vi "SetUpLeCroy930xx.vi"(6 "Therapy (T)":bool, 7 "Therapy VISA session in":refnum<visa-resource-name>, 8 "33250(T)/33120(F)":bool=TRUE, 11 "VISA session":refnum<visa-resource-name>) -> (1 "Equivalent delay\ndistance (mm)":dbl=1.5 format="%.2f", 2 "RF data Out":T2 {"Delay (micro s)" format="%.2f"})   [LabVIEW 2022 SP3]
uses:
  Motion Controllers/-MotionRoutines/MotionGlobals.vi
  <vilib>/Analysis/NI_AALPro.lvlib
  <vilib>/Utility/file.llb/Write To Spreadsheet File (DBL).vi
  <vilib>/Analysis/NI_AALBase.lvlib
  <vilib>/Analysis/baseanly.llb/Mean (DBL).vi
panel:
  in  "Grab Settings":bool
  in  "Save trace?":bool
  out "Lines in burst":i32=1 min=1 max=50000 step=1
  in  "cycles (f), time(t)":bool=TRUE
  in  "Set Panametrics":bool
  out "Scope Delay (ms)":dbl=1.5 format="%.2f"
  in  "go to scan type":bool
  in  "Therapy Burst Set Up":T1={"Therapy Set Up"={"Burst time (ms)"=1.0, "Frequency (MHz)"=1.0, "Amplitude (mV)"=10.0}, "Divide prf by"=1, "Therapy Delay (ms) "=0.0, "Turn off therapy (T)"=TRUE} {"Therapy Delay (ms)" format="%.2f"; "Therapy Set Up"."Amplitude (mV)" min=10.0 max=1000.0 format="%.2f"; "Therapy Set Up"."Frequency (MHz)" format="%.4f"; "Therapy Set Up"."Burst time (ms)" min=1 max=50000 step=1 format="%.3f"}
  in  "ExitSendCmd":bool
  out "Time scale per Div":i32(ring)=3 items=["100 ns", "200 ns", "500 ns", "1 micros", "2 micros", "5 micros", "10 micros", "20 micros", "50 micros", "100 micros", "200 micros", "500 micros", "1 ms", "2 ms", "5 ms", "10 ms", "20 ms", "50 ms", "100 ms", "200 ms"]
  out "Waveform\nGraph":cluster{i32, dbl, dbl[]}(graph)
  in  "Trigger Settings":T3={"Source"=1, "Coupling"=0, "Slope"=0, "Level (mV)"=1000.0} {"Slope" items=["Positive", "Negative"]; "Level (mV)" format="%.2f"; "Coupling" items=["DC 1 MOhm", "AC 1 MOhm", "DC 50 Ohm", "AC 50 Ohm"]; "Source" items=["Chan 1", "External"]}
  in  "RF data Sampling":T4={"Sampling Rate"=5, "Ref Delay (ms)"=0.0, "rf points per line"=2048} {"Ref Delay (ms)" format="%.2f"}
  # "Digitizer Settings"
  # "Set Up trace on Scope, then select Grab Settings to verify trace is captured."
  # "Need to autoscale if viewing spectrum. Yellow curser used for additional delay.\nRF data is captured between yellow and red lines."
  # "© 2000-2002 Riverside Research Institute"
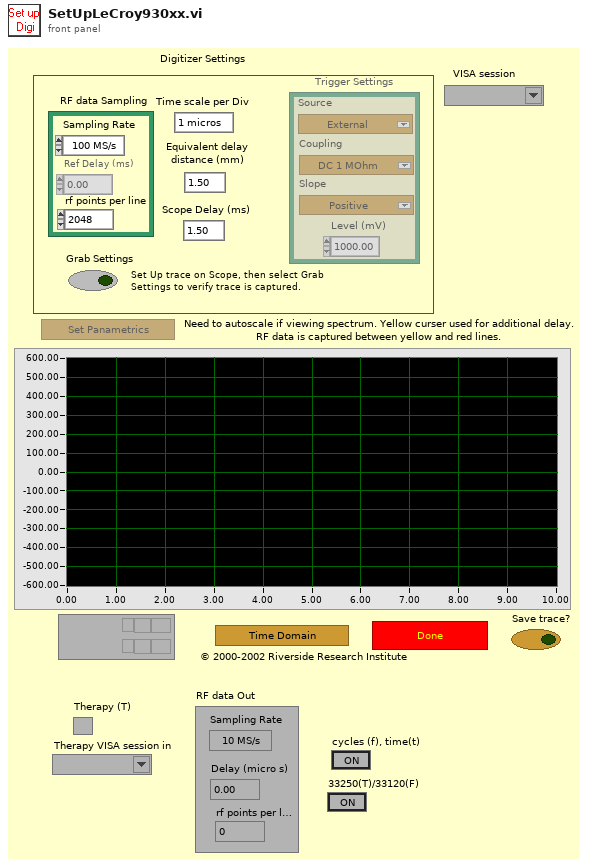
[diagram p1: front panel]
types:
  T1 = cluster{"Therapy Set Up":cluster{"Burst time (ms)":sgl, "Frequency (MHz)":dbl, "Amplitude (mV)":dbl}, "Divide prf by":i32, "Therapy Delay (ms) ":dbl, "Turn off therapy (T)":bool}
  T2 = cluster{"Sampling Rate":u16, "Delay (micro s)":dbl, "rf points per line":u16}
  T3 = cluster{"Source":u16, "Coupling":u16, "Slope":u16, "Level (mV)":dbl}
  T4 = cluster{"Sampling Rate":u16, "Ref Delay (ms)":dbl, "rf points per line":u16}
  T5 = cluster{"Burst time (ms)":sgl, "Frequency (MHz)":dbl, "Amplitude (mV)":dbl}
  T6 = cluster{"t(0) (sec)":ext, "Delta t (sec)":dbl, "Amplitude Array (Volts)":sgl[]}
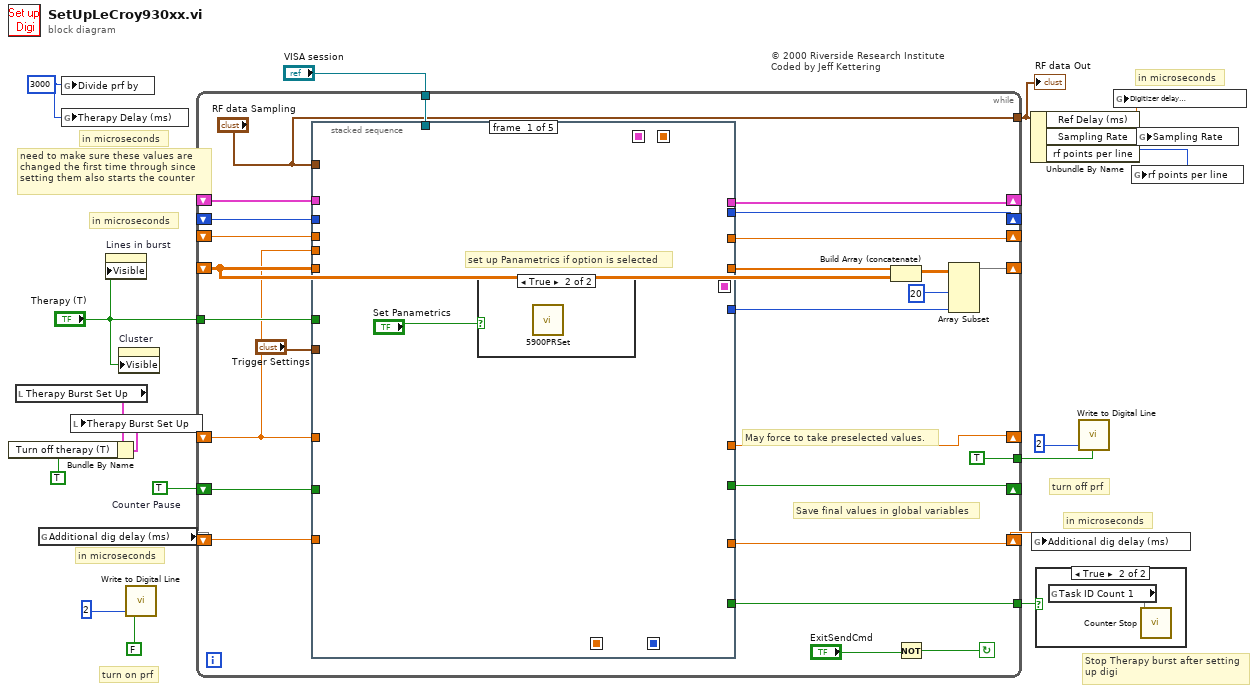
[diagram p0: block diagram]
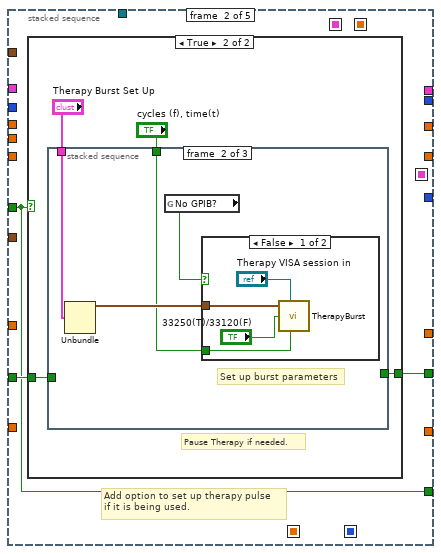
[diagram p3: hidden frame]
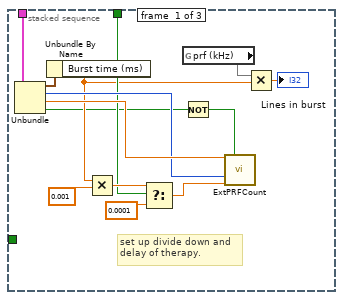
[diagram p5: hidden frame]
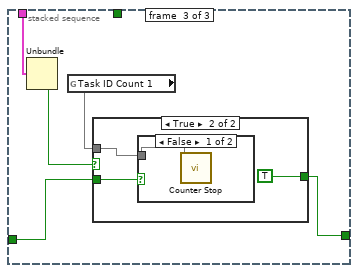
[diagram p7: hidden frame]
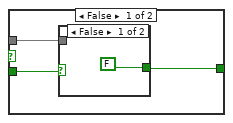
[diagram p8: hidden frame]
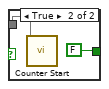
[diagram p9: hidden frame]
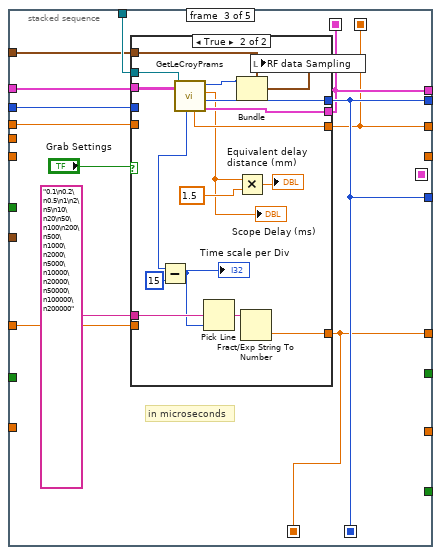
[diagram p11: hidden frame]
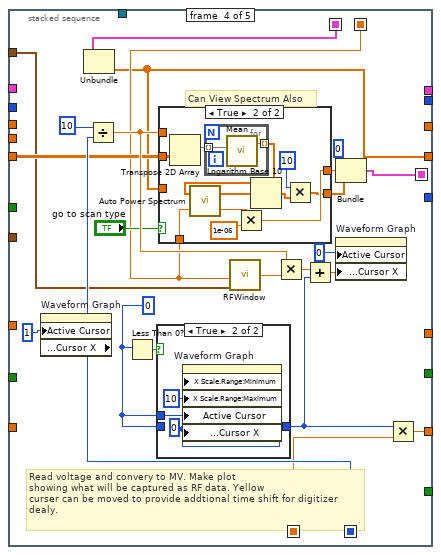
[diagram p13: hidden frame]
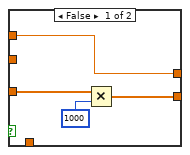
[diagram p15: hidden frame]
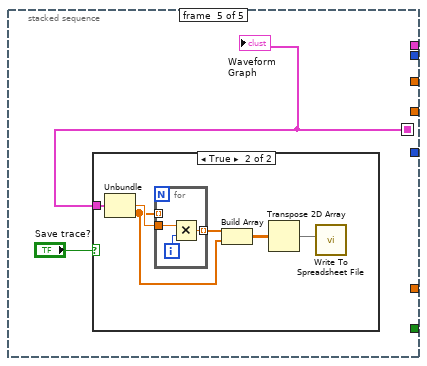
[diagram p16: hidden frame]
diagram:
  w17 = 3000
  w18 = TRUE  # Counter Pause
  # "turn on prf"
  # "turn off prf"
  # "© 2000 Riverside Research Institute\nCoded by Jeff Kettering"
  # "Stop Therapy burst after setting\nup digi"
  # "in microseconds"
  # "in microseconds"
  # "in microseconds"
  # "in microseconds"
  # "in microseconds"
  # "need to make sure these values are\nchanged the first time through since\nsetting them also starts the counter"
  n1 = local read "Therapy Burst Set Up"() -> (w10:T1)
  n2 = Bundle By Name(cluster=w10, "Turn off therapy (T)"=TRUE) -> (w9:T1)
  n3 = global read "MotionGlobals.vi" "Additional dig delay (ms)"() -> (w12)
  n4 = global write "MotionGlobals.vi" "Divide prf by"(w17) -> ()
  n5 = global write "MotionGlobals.vi" "Therapy Delay (ms)"(w17) -> ()
  n6 = local write "Therapy Burst Set Up"(w9) -> ()
  n7 = property on="Lines in burst" class="DigNum (strict)"("Visible"="Therapy (T)") -> ()  [unwired: 2 in, 2 out]
  n8 = property on="Cluster" class="Clust (strict)"("Visible"="Therapy (T)") -> ()  [unwired: 2 in, 2 out]
  n9 = call <vilib>:"Write to Digital Line.vi"("line"=2, "line state"=FALSE) -> ()  [unwired: 7 in]
  n10 = while {
    tunnel: [TRUE] -> w3
    tunnel: [w30] -> w7
    shift-left: _ -> [w35]
    shift-right: [w33] -> _
    shift-left: w12 -> [w38]
    shift-right: [w37] -> w11
    tunnel: ["RF data Sampling"] -> w14
    shift-left: w18 -> [w40]
    shift-right: [w39] -> _
    tunnel: "Therapy (T)" -> [w41]
    tunnel: "VISA session" -> [w28]
    shift-right: [w26] -> _
    shift-left: _ -> [w24]
    shift-right: [w27] -> _
    shift-left: _ -> [w22]
    shift-right: [w25] -> _
    shift-left: _ -> [w23]
    shift-right: [w20] -> _
    shift-left: _ -> [w21]
    stop <- w42 continue-if-true
    # "May force to take preselected values."
    # "Save final values in global variables"
    n11 = stacked-sequence {
      seq-local: [_ _ w99 _ _] -> [_ _ _ w141 _]
      seq-local: [_ _ w92 _ _] -> [_ _ _ w137 _]
      seq-local: [_ _ _ w128 _] -> [_ _ _ _ w167]
      seq-local: [_ _ w98 _ _] -> [_ _ _ w126 _]
      seq-local: [_ _ w97 _ _] -> [_ _ _ w127 _]
      tunnel: "RF data Sampling" -> [_ _ w91 w130 _]
      tunnel: "Trigger Settings" -> [_ _ _ _ _]
      tunnel: w41 -> [_ w46 _ _ _]
      tunnel: w40 -> [_ w48 _ _ _]
      tunnel: [_ w47 _ _ _] -> w39
      tunnel: w38 -> [_ _ _ _ _]
      tunnel: [_ _ _ w129 _] -> w37
      tunnel: w35 -> [_ _ _ w132 _]
      tunnel: [_ _ _ w125 _] -> w36
      tunnel: [_ _ w99 _ _] -> w32
      tunnel: [_ w46 _ _ _] -> w30
      tunnel: w28 -> [_ _ w101 _ _]
      tunnel: [_ _ w99 _ _] -> w27
      tunnel: [_ _ w98 _ _] -> w26
      tunnel: [_ _ w97 _ _] -> w25
      tunnel: w24 -> [_ _ w96 _ _]
      tunnel: w23 -> [_ _ w95 _ _]
      tunnel: w22 -> [_ _ w94 _ _]
      tunnel: w21 -> [_ _ _ _ _]
      tunnel: [_ _ w92 _ _] -> w20
      tunnel: w21 -> [_ _ w93 _ _]
      frame #0 {
        # "set up Panametrics if option is selected"
        n12 = case shown="True" "Set Panametrics" {
          frame False {
          }
          frame True {
            n13 = call "5900PRSet.vi"() -> ()  [unwired: 13 in, 3 out]
          }
        }
      }
      frame #1 {
        # "Add option to set up therapy pulse\nif it is being used."
        n14 = case shown="True" w46 {
          tunnel: w48 -> [w49 w52]
          tunnel: [w49 w51] -> w47
          frame False {
          }
          frame True {
            # "Pause Therapy if needed."
            n15 = stacked-sequence {
              tunnel: "Therapy Burst Set Up" -> [w59 w71 w77]
              tunnel: w52 -> [_ _ w79]
              tunnel: [_ _ w78] -> w51
              tunnel: "cycles (f), time(t)" -> [w58 w68 _]
              frame #0 {
                # "set up divide down and\ndelay of therapy."
                n16 = Unbundle(w59) -> ("Therapy Set Up"=w65:T5, "Divide prf by"=w66:i32, "Therapy Delay (ms)"=w67:dbl, "Turn off therapy (T)"=w55:bool)
                n17 = Unbundle By Name(w65) -> ("Burst time (ms)"=w57:sgl)
                n18 = Multiply(x=w57, y=0.001) -> (x*y=w62:dbl)
                n19 = Select(t=w62, s=w58, f=0.0001) -> (s? t:f=w64:dbl)
                n20 = global read "MotionGlobals.vi" "prf (kHz)"() -> (w60)
                n21 = Not(x=w55) -> (.not. x?=w54:bool)
                n22 = call "ExtPRFCount.vi"("Therapy Delay (ms)"=w67, "Start Counter?"=w54, "Divide prf by"=w66, "pulse width (s or cycles)"=w64) -> ()  [unwired: 10 in, 2 out]
                n23 = Multiply(x=w60, y=w57) -> (x*y=→"Lines in burst":sgl)
              }
              frame #1 {
                # "Set up burst parameters"
                n24 = Unbundle(w71) -> ("Therapy Set Up"=w70:T5)  [unwired: 3 out]
                n25 = global read "MotionGlobals.vi" "No GPIB?"() -> (w69:bool)
                n26 = case shown="False" w69 {
                  tunnel: w70 -> [w75 _]
                  tunnel: w68 -> [w74 _]
                  frame False {
                    n27 = call "TherapyBurst.vi"("Input Cluster"=w75, "VISA session in"="Therapy VISA session in", "33250(T)/33120(F)"="33250(T)/33120(F)", "Trigger (F) Gate(T)"=w74) -> ()  [unwired: 2 in, 3 out]
                  }
                  frame True {
                  }
                }
              }
              frame #2 {
                n28 = Unbundle(w77) -> ("Turn off therapy (T)"=w76:bool)  [unwired: 3 out]
                n29 = global read "MotionGlobals.vi" "Task ID Count 1"() -> (w80)
                n30 = case shown="True" w76 {
                  tunnel: w80 -> [w82 w89]
                  tunnel: w79 -> [w83 w87]
                  tunnel: [w81 TRUE] -> w78
                  frame False {
                    n31 = case shown="False" w83 {
                      tunnel: [FALSE FALSE] -> w81
                      tunnel: w82 -> [_ w85]
                      frame False {
                      }
                      frame True {
                        n32 = call <vilib>:"Counter Start.vi"("taskID"=w85) -> ()  [unwired: 9 in, 2 out]
                      }
                    }
                  }
                  frame True {
                    n33 = case shown="False" w87 {
                      tunnel: w89 -> [w90 _]
                      frame False {
                        n34 = call <vilib>:"Counter Stop.vi"("taskID"=w90) -> ()  [unwired: 5 in, 2 out]
                      }
                      frame True {
                      }
                    }
                  }
                }
              }
            }
          }
        }
      }
      frame #2 {
        # "in microseconds"
        n35 = case shown="True" "Grab Settings" {
          tunnel: w101 -> [_ w122]
          tunnel: [w106 w121] -> w98
          tunnel: [w104 w120] -> w99
          tunnel: [w105 w115] -> w97
          tunnel: w96 -> [w106 _]
          tunnel: w95 -> [w105 _]
          tunnel: w94 -> [w104 _]
          tunnel: "0.1\n0.2\n0.5\n1\n2\n5\n10\n20\n50\n100\n200\n500\n1000\n2000\n5000\n10000\n20000\n50000\n100000\n200000" ("ResourceName") -> [_ w112]
          tunnel: [w103 w110] -> w92
          tunnel: w93 -> [w103 _]
          tunnel: w91 -> [_ w108]
          frame False {
          }
          frame True {
            n36 = call "GetLeCroyPrams.vi"("VISA session"=w122) -> ("Waveform Graph"=w121:T6, "RF PTS"=w120:i32, "Delay (micros)"=w114:dbl, "Sampling Rate"=w109:u16, "sampling time"=w115:sgl, "TIMEBASE"=w119:i16)  [unwired: 4 in, 1 out]
            "Scope Delay (ms)" <- w114
            n37 = Subtract(x=w119, y=15) -> (x-y=w111:i32)
            "Time scale per Div" <- w111
            n38 = Pick Line(multi-line string=w112, line index=w111) -> (output string=w113:string)  [unwired: 1 in]
            n39 = Bundle(cluster=w108, "Sampling Rate"=w109) -> (w107:T4)  [unwired: 2 in]
            n40 = Multiply(x=w114, y=1.5) -> (x*y=→"Equivalent delay\ndistance (mm)":dbl)
            n41 = Fract/Exp String To Number(string=w113) -> (number=w110:dbl)  [unwired: 3 in, 1 out]
            n42 = local write "RF data Sampling"(w107) -> ()
          }
        }
      }
      frame #3 {
        w123 = 0
        # "Can View Spectrum Also"
        # "Read voltage and convery to MV. Make plot\nshowing what will be captured as RF data. Yellow\ncurser can be moved to provide addtional time shift for digitizer\ndealy."
        n43 = property on="Waveform Graph" class="WFGraph (strict)" props=["Active Cursor", "Cursor", "Cursor Position:Cursor X"]("Active Cursor"=u32 1 ("Write Attribute")) -> ()  [unwired: 2 in, 3 out]
        n44 = Unbundle(w126) -> ("Amplitude Array (Volts)"=w125:sgl[])  [unwired: 2 out]
        n45 = Divide(x=10, y=w141) -> (x/y=w140:dbl)
        n46 = Less Than 0?(x=w123) -> (x < 0?=w133:bool)
        n47 = case shown="True" w133 {
          tunnel: w123 -> [w146 _]
          tunnel: [w146 w147] -> w135
          tunnel: w123 -> [_ w149]
          frame False {
          }
          frame True {
            w147 = 0
            n48 = property on="Waveform Graph" class="WFGraph (strict)"("X Scale.Range:Minimum"=w147, "X Scale.Range:Maximum"=10, "Active Cursor"=w149, "Cursor.Cursor Position:Cursor X"=w147) -> ()  [unwired: 2 in, 2 out]
          }
        }
        n49 = case shown="True" "go to scan type" {
          tunnel: [w152 w156] -> w131
          tunnel: w125 -> [w151 _]
          tunnel: [w150 w161] -> w139
          tunnel: w140 -> [w150 _]
          tunnel: w132 -> [_ w159]
          tunnel: w127 -> [_ w154]
          frame False {
            n50 = Multiply(x=w151, y=1000) -> (x*y=w152:sgl[])
          }
          frame True {
            n51 = Transpose 2D Array(2D array=w159) -> (transposed array=w158:sgl[][])
            n52 = for {
              tunnel: w158 -> [w166] mode=indexing
              tunnel: [w165] -> w157 mode=indexing
              n53 = call-poly <vilib>:"Mean.vi"("X"=w166) -> ("mean"=w165:dbl)  [unwired: 1 out]
            }
            n54 = call <vilib>:"Auto Power Spectrum.vi"("dt"=w154, "Signal (V)"=w157) -> ("df"=w163:dbl, "Power Spectrum (V^2 rms)"=w164:dbl[])
            n55 = Multiply(x=w163, y=1e-06) -> (x*y=w161:dbl)
            n56 = Logarithm Base 10(1:w164) -> (0:w160:dbl[])
            n57 = Multiply(x=10, y=w160) -> (x*y=w156:dbl[])
          }
        }
        n58 = call "RFWindow.vi"("RF data Sampling"=w130, "Sample Time"=w127) -> ("curser position"=w142:dbl)  [unwired: 2 in]
        n59 = Multiply(x=w140, y=w142) -> (x*y=w136:dbl)
        n60 = Add(x=w136, y=w135) -> (x+y=w134:dbl)
        n61 = Bundle(0, w139, w131) -> (w128:cluster{i32, dbl, dbl[]})  [unwired: 1 in]
        n62 = property on="Waveform Graph" class="WFGraph (strict)"("Active Cursor"=0, "Cursor.Cursor Position:Cursor X"=w134) -> ()  [unwired: 2 in, 2 out]
        n63 = Multiply(x=w135, y=w137) -> (x*y=w129:dbl)
      }
      frame #4 {
        n64 = case shown="True" "Save trace?" {
          tunnel: w167 -> [_ w174]
          frame False {
          }
          frame True {
            n65 = Unbundle(w174) -> (w173:dbl, w171:dbl[])  [unwired: 1 out]
            n66 = for {
              tunnel: w173 -> [w176]
              tunnel: w171 -> [_] mode=indexing
              tunnel: [w175] -> w172 mode=indexing
              i -> [w177]
              n67 = Multiply(x=w176, y=w177) -> (x*y=w175:dbl)
            }
            n68 = Build Array(w172, w171) -> (w170:dbl[][])
            n69 = Transpose 2D Array(2D array=w170) -> (transposed array=w169:dbl[][])
            n70 = call-poly <vilib>:"Write To Spreadsheet File.vi"("2D data"=w169) -> ()  [unwired: 7 in, 1 out]
          }
        }
        "Waveform\nGraph" <- w167
      }
    }
    n71 = Build Array (concatenate)(w36, w35) -> (w34:sgl[][])
    n72 = Not(x="ExitSendCmd") -> (.not. x?=w42:bool)
    n73 = Array Subset(array=w34, length (row)=20, length (col)=w32) -> (w33:sgl[][])  [unwired: 2 in]
  }
  "RF data Out" <- w14
  n74 = Unbundle By Name(w14) -> ("Ref Delay (ms)"=w16:dbl, "Sampling Rate"=w15:u16, "rf points per line"=w13:u16)
  n75 = global write "MotionGlobals.vi" "Additional dig delay (ms)"(w11) -> ()
  n76 = case shown="True" w7 {
    frame False {
    }
    frame True {
      n77 = global read "MotionGlobals.vi" "Task ID Count 1"() -> (w178)
      n78 = call <vilib>:"Counter Stop.vi"("taskID"=w178) -> ()  [unwired: 5 in, 2 out]
    }
  }
  n79 = call <vilib>:"Write to Digital Line.vi"("line"=2, "line state"=w3) -> ()  [unwired: 7 in]
  n80 = global write "MotionGlobals.vi" "Digitizer delay\n (ms)"(w16) -> ()
  n81 = global write "MotionGlobals.vi" "rf points per line"(w13) -> ()
  n82 = global write "MotionGlobals.vi" "Sampling Rate"(w15) -> ()
